vi "move_crystal_to_position.vi"(7 "Crystal Speed / counts s-1":dbl, 8 "error in":errorcluster, 9 "Desired Position":i32, 10 "Crystal Number":u16(ring) items=["Crystal 1", "Crystal 2", "Crystal 3", "Crystal 4", "Crystal 5", "Crystal 6", "Crystal 7", ""], 11 "address":string) -> (0 "error out":errorcluster, 2 "Crystal Number Out":i32)   [LabVIEW 2020]
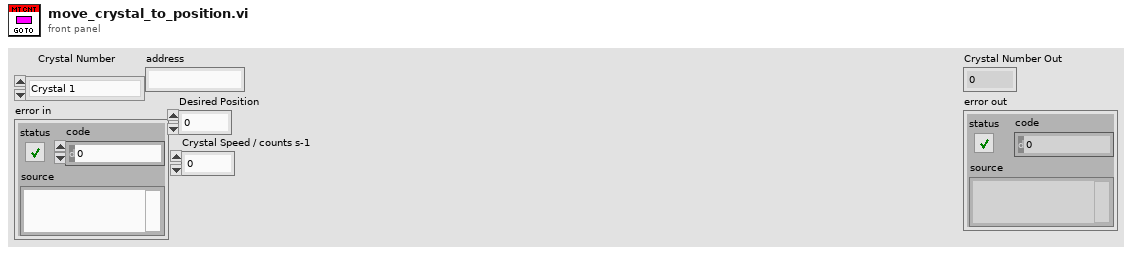
[diagram p1: front panel]
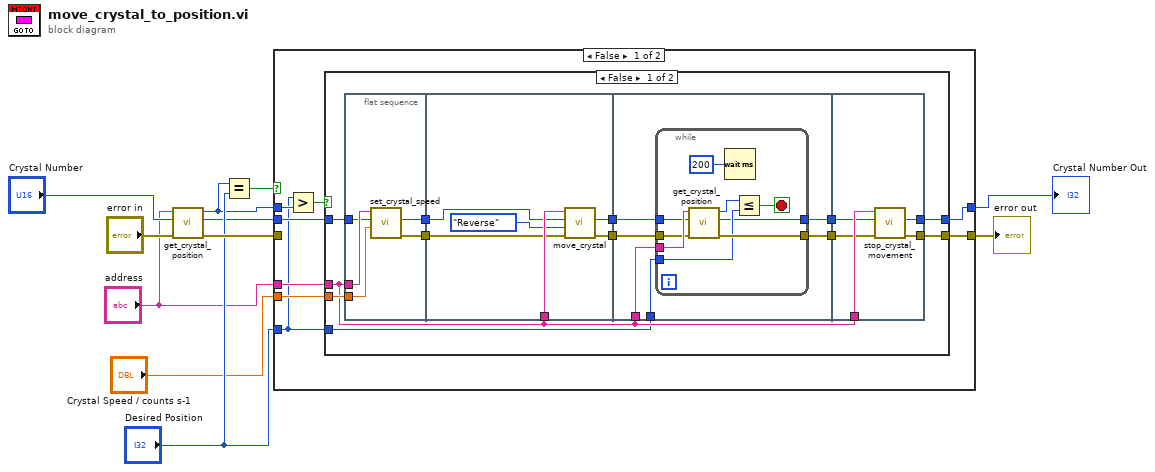
[diagram p0: block diagram]
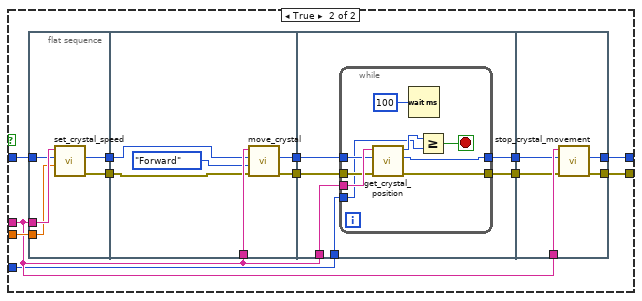
[diagram p2: hidden frame]
diagram:
  n1 = call "get_crystal_position.vi"("error in"="error in", "Crystal Number"="Crystal Number", "address"="address") -> ("error out"=w8:errorcluster, "Crystal Number Out"=w5:u16, "Crystal Position"=w4:i32)  [unwired: 6 in]
  n2 = Equal?(x=w4, y="Desired Position") -> (x = y?=w9:bool)
  n3 = case shown="False" w9 {
    tunnel: w8 -> [_ w107]
    tunnel: [w14 w107] -> w1
    tunnel: "Desired Position" -> [w12 _]
    tunnel: "address" -> [w18 _]
    tunnel: w5 -> [w17 _]
    tunnel: w4 -> [w15 w106]
    tunnel: "Crystal Speed / counts s-1" -> [w16 _]
    tunnel: [w13 w106] -> w2
    frame False {
      n4 = Greater?(x=w12, y=w15) -> (0:w19:bool)
      n5 = case shown="False" w19 {
        tunnel: w18 -> [w22 w68]
        tunnel: w17 -> [w24 w74]
        tunnel: w16 -> [w23 w69]
        tunnel: [w25 w65] -> w14
        tunnel: [w26 w64] -> w13
        tunnel: w12 -> [w21 w63]
        frame False {
          n6 = flat-sequence {
            tunnel: w22 -> [w36]
            tunnel: w24 -> [w35]
            tunnel: [w34] -> w31
            tunnel: [w33] -> w30
            tunnel: w23 -> [w32]
            tunnel: w22 -> [w42]
            tunnel: w31 -> [w41]
            tunnel: [w40] -> w29
            tunnel: w30 -> [w39]
            tunnel: [w38] -> w28
            tunnel: w22 -> [w48]
            tunnel: w29 -> [w47]
            tunnel: w28 -> [w46]
            tunnel: [w45] -> w27
            tunnel: w21 -> [w44]
            tunnel: [w43] -> w20
            tunnel: w22 -> [w62]
            tunnel: w27 -> [w61]
            tunnel: [w60] -> w25
            tunnel: [w59] -> w26
            tunnel: w20 -> [w58]
            frame #0 {
              n7 = call "set_crystal_speed.vi"("Crystal Speed / counts s-1"=w32, "Crystal Number"=w35, "address"=w36) -> ("error out"=w33:errorcluster, "Crystal Number Out"=w34:u16)  [unwired: 7 in]
            }
            frame #1 {
              n8 = call "move_crystal.vi"("error in"=w39, "Direction"=enum16{"Reverse", "Forward"}."Reverse", "Crystal Number"=w41, "address"=w42) -> ("error out"=w40:errorcluster, "Crystal Number Out"=w38:u16)  [unwired: 6 in]
            }
            frame #2 {
              n9 = while {
                tunnel: w48 -> [w57]
                tunnel: w47 -> [w56]
                tunnel: w46 -> [w55]
                tunnel: [w52] -> w45
                tunnel: w44 -> [w50]
                tunnel: [w49] -> w43
                stop <- w53 stop-if-true
                n10 = call "get_crystal_position.vi"("error in"=w56, "Crystal Number"=w55, "address"=w57) -> ("error out"=w52:errorcluster, "Crystal Number Out"=w49:u16, "Crystal Position"=w51:i32)  [unwired: 6 in]
                n11 = Wait (ms)(milliseconds to wait=u32 200) -> ()  [unwired: 1 out]
                n12 = Less Or Equal?(x=w51, y=w50) -> (x <= y?=w53:bool)
              }
            }
            frame #3 {
              n13 = call "stop_crystal_movement.vi"("error in"=w61, "Crystal Number"=w58, "address"=w62) -> ("error out"=w60:errorcluster, "Crystal Number Out"=w59:u16)  [unwired: 7 in]
            }
          }
        }
        frame True {
          n14 = flat-sequence {
            tunnel: w68 -> [w79]
            tunnel: w74 -> [w78]
            tunnel: [w77] -> w73
            tunnel: [w76] -> w71
            tunnel: w69 -> [w75]
            tunnel: w68 -> [w85]
            tunnel: w73 -> [w84]
            tunnel: [w83] -> w72
            tunnel: w71 -> [w82]
            tunnel: [w81] -> w70
            tunnel: w68 -> [w91]
            tunnel: w72 -> [w90]
            tunnel: w70 -> [w89]
            tunnel: w63 -> [w88]
            tunnel: [w87] -> w67
            tunnel: [w86] -> w66
            tunnel: w68 -> [w105]
            tunnel: w67 -> [w104]
            tunnel: w66 -> [w103]
            tunnel: [w102] -> w65
            tunnel: [w101] -> w64
            frame #0 {
              n15 = call "set_crystal_speed.vi"("Crystal Speed / counts s-1"=w75, "Crystal Number"=w78, "address"=w79) -> ("error out"=w76:errorcluster, "Crystal Number Out"=w77:u16)  [unwired: 7 in]
            }
            frame #1 {
              n16 = call "move_crystal.vi"("error in"=w82, "Direction"=enum16{"Reverse", "Forward"}."Forward", "Crystal Number"=w84, "address"=w85) -> ("error out"=w83:errorcluster, "Crystal Number Out"=w81:u16)  [unwired: 6 in]
            }
            frame #2 {
              n17 = while {
                tunnel: w91 -> [w100]
                tunnel: w90 -> [w99]
                tunnel: w89 -> [w98]
                tunnel: w88 -> [w95]
                tunnel: [w93] -> w87
                tunnel: [w92] -> w86
                stop <- w94 stop-if-true
                n18 = call "get_crystal_position.vi"("error in"=w99, "Crystal Number"=w98, "address"=w100) -> ("error out"=w92:errorcluster, "Crystal Number Out"=w93:u16, "Crystal Position"=w96:i32)  [unwired: 6 in]
                n19 = Wait (ms)(milliseconds to wait=u32 100) -> ()  [unwired: 1 out]
                n20 = Greater Or Equal?(x=w96, y=w95) -> (x >= y?=w94:bool)
              }
            }
            frame #3 {
              n21 = call "stop_crystal_movement.vi"("error in"=w103, "Crystal Number"=w104, "address"=w105) -> ("error out"=w102:errorcluster, "Crystal Number Out"=w101:u16)  [unwired: 7 in]
            }
          }
        }
      }
    }
    frame True {
    }
  }
  "Crystal Number Out" <- w2
  "error out" <- w1
